vi "RSZVB Start Calibration With Options.vi"(0 "VISA session":refnum<visa-resource-name>, 1 "Dispersion (F: Off)":bool, 2 "Delay/Phase Value (0.0)":dbl format="%^.3e", 5 "Channel (1)":i32=1, 7 "Standard (0: Unknown Through)":i32(ring) items=["Unknown Through"], 9 "Port 1 (1)":i32=1, 11 "error in (no error)":errorcluster {"code" format="%.0x"}, 12 "Delay/Phase (0: Auto)":i32(ring) items=["Auto", "Manual"], 13 "Port 2 (1)":i32=1) -> (4 "dup VISA session":refnum<visa-resource-name>, 15 "error out":errorcluster {"code" format="%.0x"})   [LabVIEW 2011]
doc: "This VI starts a calibration measurement in order to acquire measurement data for the selected standards. The\nstandards are reflection or transmission standards and can be connected to arbitrary analyzer ports.\n\nNote(s):\n\n(1) For some measurements the default set timeout can be insufficient. To set higher timeout use VI rszvb_setTimeOut.\n\n(2) This VI is available with firmware version 2.40 and higher.\n\nRemote-control command(s):\n[SENSe<Ch>:]CORRection:COLLect[:ACQuire]:SELected UTHRough,<port_no>,<port_no>[,<Dispersion>,AUTO | <delay | phase>]"
uses:
  _utility/RSZVB Global Data.vi
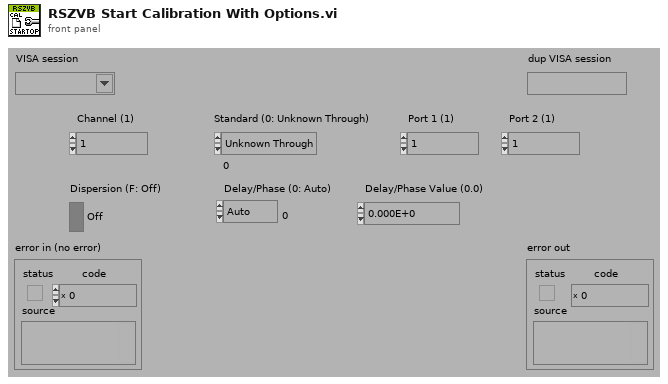
[diagram p1: front panel]
types:
  T1 = cluster{"Error Checking (T: On)":bool, "Installed Options":string[], "Data Valid?":bool, "Ports":i32, "Model":string[], "Option Checking (T: On)":bool}[]
  T2 = cluster{"Error Checking (T: On)":bool, "Installed Options":string[], "Data Valid?":bool, "Ports":i32, "Model":string[], "Option Checking (T: On)":bool}
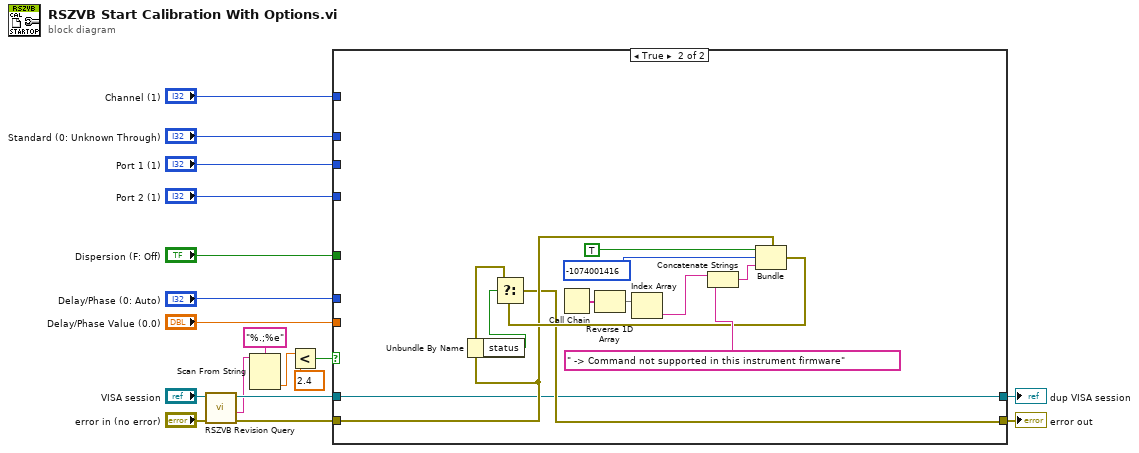
[diagram p0: block diagram]
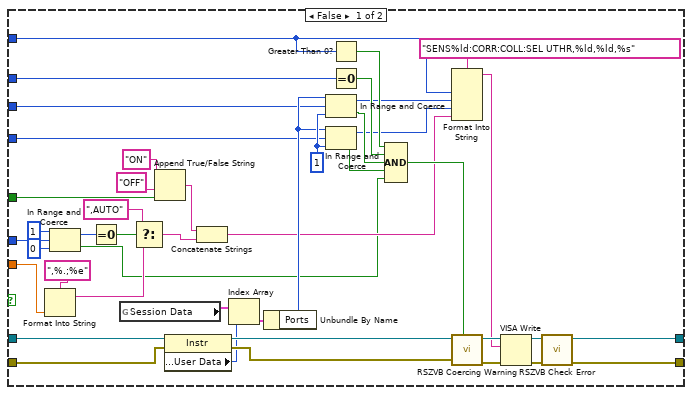
[diagram p2: hidden frame]
diagram:
  n1 = call "RSZVB Revision Query.vi"("error in (no error)"="error in (no error)", "VISA session"="VISA session") -> ("error out"=w7:errorcluster, "Instrument Firmware Revision"=w2:string, "dup VISA session"=w6:refnum<visa-resource-name>)  [unwired: 6 in, 1 out]
  n2 = Scan From String(format string="%.;%e", input string=w2) -> (output 1=w4:dbl)  [unwired: 3 in, 3 out]
  n3 = Less?(x=w4, y=2.4) -> (x < y?=w1:bool)
  n4 = case shown="True" w1 {
    tunnel: "Channel (1)" -> [w52 _]
    tunnel: "Standard (0: Unknown Through)" -> [w51 _]
    tunnel: "Port 1 (1)" -> [w47 _]
    tunnel: "Port 2 (1)" -> [w46 _]
    tunnel: "Dispersion (F: Off)" -> [w36 _]
    tunnel: "Delay/Phase Value (0.0)" -> [w19 _]
    tunnel: [w28 w63] -> w12
    tunnel: [w27 w64] -> w11
    tunnel: "Delay/Phase (0: Auto)" -> [w26 _]
    tunnel: w7 -> [w21 w65]
    tunnel: w6 -> [w20 w63]
    frame False {
      w49 = 1 ("lower limit")
      n5 = Format Into String(format string=",%.;%e", w19) -> (resulting string=w33:string)  [unwired: 2 in, 1 out]
      n6 = In Range and Coerce(upper limit=1, x=w26, lower limit=0) -> (coerced(x)=w23:i32, In Range?=w22:bool)
      n7 = Equal To 0?(x=w23) -> (x = 0?=w39:bool)
      n8 = global read "RSZVB Global Data.vi" "Session Data"() -> (w57:T1)
      n9 = Select(t=",AUTO" ("true string"), s=w39, f=w33) -> (s? t:f=w31:string)
      n10 = Append True/False String(1:w36, 2:"OFF" ("false string"), 3:"ON" ("true string")) -> (0:w32:string)  [unwired: 1 in]
      n11 = property class="Instr"(reference=w20, error in=w21) -> (reference out=w55:refnum<visa-resource-name>, error out=w56:errorcluster, "General Settings:User Data"=w54:u32)
      n12 = Concatenate Strings(w32, w31) -> (w30:string)
      n13 = Index Array(array=w57, index=w54) -> (element=w58:T2)
      n14 = Unbundle By Name(w58) -> ("Ports"=w48:i32)
      n15 = In Range and Coerce(upper limit=w48, x=w47, lower limit=w49) -> (coerced(x)=w41:i32, In Range?=w44:bool)
      n16 = In Range and Coerce(upper limit=w48, x=w46, lower limit=w49) -> (coerced(x)=w40:i32, In Range?=w45:bool)
      n17 = Greater Than 0?(x=w52) -> (x > 0?=w42:bool)
      n18 = Equal To 0?(x=w51) -> (x = 0?=w43:bool)
      n19 = Compound Arithmetic op=AND(w42, w43, w44, w45, w22) -> (w53:bool)
      n20 = Format Into String(format string="SENS%ld:CORR:COLL:SEL UTHR,%ld,%ld,%s", w52, w41, w40, w30) -> (resulting string=w29:string)  [unwired: 2 in, 1 out]
      n21 = call "RSZVB Coercing Warning.vi"("In Range?"=w53, "error in (no error)"=w56, "VISA session"=w55) -> ("error out"=w60:errorcluster, "dup VISA session"=w59:refnum<visa-resource-name>)  [unwired: 7 in]
      n22 = VISA Write(VISA resource name=w59, write buffer=w29, error in (no error)=w60) -> (VISA resource name out=w61:refnum<visa-resource-name>, error out=w62:errorcluster)  [unwired: 1 out]
      n23 = call "RSZVB Check Error.vi"("error in (no error)"=w62, "VISA session"=w61) -> ("error out"=w27:errorcluster, "dup VISA session"=w28:refnum<visa-resource-name>)  [unwired: 8 in]
    }
    frame True {
      n24 = Unbundle By Name(w65) -> ("status"=w67:bool)
      n25 = Call Chain() -> (call chain=w70:string[])
      n26 = Reverse 1D Array(array=w70) -> (reversed array=w71:string[])
      n27 = Index Array(array=w71) -> (element=w72:string)  [unwired: 1 in]
      n28 = Concatenate Strings(w72, " -> Command not supported in this instrument firmware" ("string")) -> (w74:string)
      n29 = Bundle(cluster=w65, "status"=TRUE, "code"=-1074001416, "source"=w74) -> (w66:errorcluster)
      n30 = Select(t=w65, s=w67, f=w66) -> (s? t:f=w64:errorcluster)
    }
  }
  "error out" <- w11
  "dup VISA session" <- w12
